vi "Interupt Example 1.vi"(8 "error in":errorcluster) -> (0 "error out":errorcluster)   [LabVIEW 2014]
doc: "Example usage of interrupts with global variables as counters. Show how to use global variables (same way as in LabVIEW)."
uses:
  <vilib>/LabVIEW Universal Transcriptor/LabVIEW to Arduino Transcriptor/Transcriptors/System API/Serial println string.vi
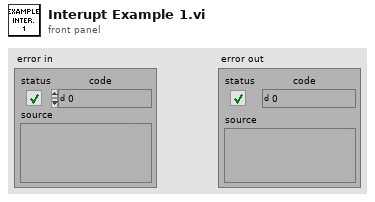
[diagram p1: front panel]
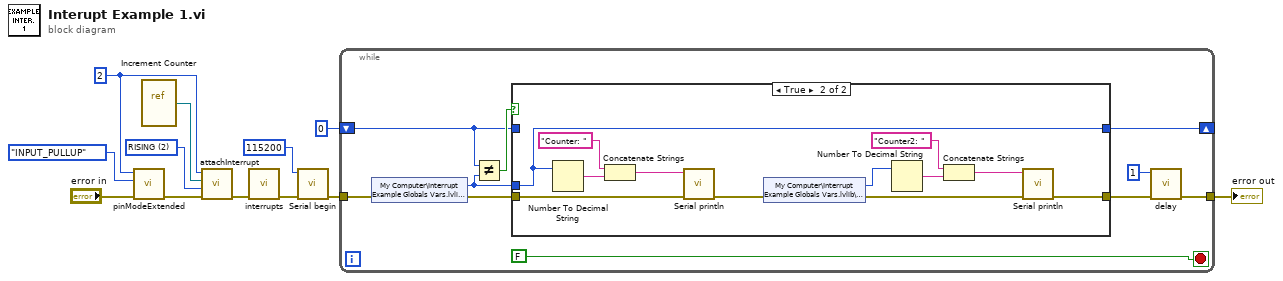
[diagram p0: block diagram]
diagram:
  w10 = u16 2 items=["LOW", "CHANGE", "RISING", "FALLING", "HIGH"] ("mode")
  w2 = 2 ("pin number")
  n1 = call <vilib>:"pinModeExtended.vi"("Error In"="error in", "mode"=enum16{"INPUT", "OUTPUT", "INPUT_PULLUP"}."INPUT_PULLUP", "pin number"=w2) -> ("Error Out"=w4:errorcluster)  [unwired: 8 in]
  n2 = vi-ref "Increment Counter.vi"() -> (w11:refnum<vi>)
  n3 = call <vilib>:"attachInterrupt.vi"("Error In"=w4, "mode"=w10, "VI Refnum"=w11, "pin number"=w2) -> ("Error Out"=w12:errorcluster)  [unwired: 7 in]
  n4 = call <vilib>:"interrupts.vi"("Error In"=w12) -> ("Error Out"=w7:errorcluster)  [unwired: 10 in]
  n5 = call <vilib>:"Serial begin.vi"("Error In"=w7, "speed (Bd)"=115200) -> ("Error Out"=w8:errorcluster)  [unwired: 9 in]
  n6 = while {
    tunnel: w8 -> [w21]
    shift-right: [w18] -> _
    shift-left: 0 ("intCounter") -> [w19]
    tunnel: [w15] -> w5
    stop <- FALSE stop-if-true
    n7 = shared-variable "My Computer\\Interrupt Example Globals Vars.lvlib\\intCounter"(error in=w21) -> (w13:i32, error out=w17:errorcluster)
    n8 = Not Equal?(x=w19, y=w13) -> (x != y?=w20:bool)
    n9 = case shown="True" w20 {
      tunnel: w19 -> [w24 _]
      tunnel: [w24 w33] -> w18
      tunnel: w17 -> [w23 w32]
      tunnel: [w23 w25] -> w16
      tunnel: w13 -> [_ w33]
      frame False {
      }
      frame True {
        n10 = Number To Decimal String(number=w33) -> (decimal integer string=w36:string)  [unwired: 1 in]
        n11 = Concatenate Strings("Counter: " ("string"), w36) -> (w34:string)
        n12 = call-poly <vilib>:"Serial println.vi"("Error In"=w32, "string in"=w34) -> ("Error Out"=w31:errorcluster)  [unwired: 9 in]
        n13 = shared-variable "My Computer\\Interrupt Example Globals Vars.lvlib\\intCounter2"(error in=w31) -> (w27:i32, error out=w26:errorcluster)
        n14 = Number To Decimal String(number=w27) -> (decimal integer string=w28:string)  [unwired: 1 in]
        n15 = Concatenate Strings("Counter2: " ("string"), w28) -> (w30:string)
        n16 = call-poly <vilib>:"Serial println.vi"("Error In"=w26, "string in"=w30) -> ("Error Out"=w25:errorcluster)  [unwired: 9 in]
      }
    }
    n17 = call <vilib>:"delay.vi"("Error In"=w16, "time (ms)"=1) -> ("Error Out"=w15:errorcluster)  [unwired: 9 in]
  }
  "error out" <- w5
